vi "Close_conn.vi"(10 "Conn":T1) -> ()   [LabVIEW 2014]
uses:
  ConsCluster.ctl
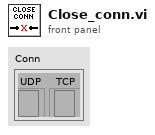
[diagram p1: front panel]
types:
  T1 = typedef "ConsCluster.ctl" = cluster{"UDP":refnum<k16>, "TCP":refnum<k5>}
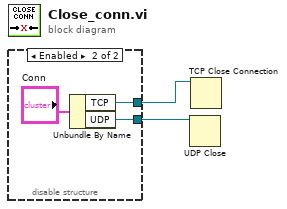
[diagram p0: block diagram]
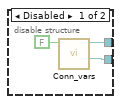
[diagram p2: hidden frame]
diagram:
  n1 = disable-structure shown="Enabled" {
    disable-tunnel: [w5 w6] -> w2
    disable-tunnel: [w4 w7] -> w1
    frame Disabled {
      n2 = call "Conn_vars.vi"("WriteVars?"=FALSE) -> ("UDPConnOut"=w4:refnum<k16>, "TCPConnOut"=w5:refnum<k5>)  [unwired: 8 in, 1 out]
    }
    frame Enabled {
      n3 = Unbundle By Name("Conn") -> ("TCP"=w6:refnum<k5>, "UDP"=w7:refnum<k16>)
    }
  }
  n4 = UDP Close(connection ID=w1) -> ()  [unwired: 1 in, 2 out]
  n5 = TCP Close Connection(connection ID=w2) -> ()  [unwired: 2 in, 2 out]
